vi "Dashboard Push.vi"() -> ()   [LabVIEW 2018]
uses:
  <vilib>/Rock Robotics/WPI/Joystick/WPI_JoystickDevRef.ctl
  <vilib>/Rock Robotics/WPI/Joystick/WPI_JoystickDeviceEnum.ctl
  b7084bc7-1634-490a-a06e-4582ec5dc279.vi
  Robot States.vi
  <vilib>/Rock Robotics/Network Tables/NT Write Boolean.vi
  Sensor Readings.vi
  Robot Global Data.vi
panel:
  in  "Joystick 0 Ref":T1
  in  "Joystick 1 Ref":T1
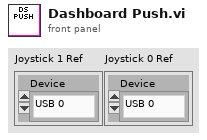
[diagram p1: front panel]
types:
  T1 = typedef "WPI_JoystickDevRef.ctl" = cluster{"Device":T2}
  T2 = typedef "WPI_JoystickDeviceEnum.ctl" = enum16{"USB 0", "USB 1", "USB 2", "USB 3", "USB 4", "USB 5"}
  T3 = cluster{"[0]":bool, "[1]":bool, "[2]":bool, "[3]":bool, "[4]":bool, "[5]":bool, "[6]":bool}
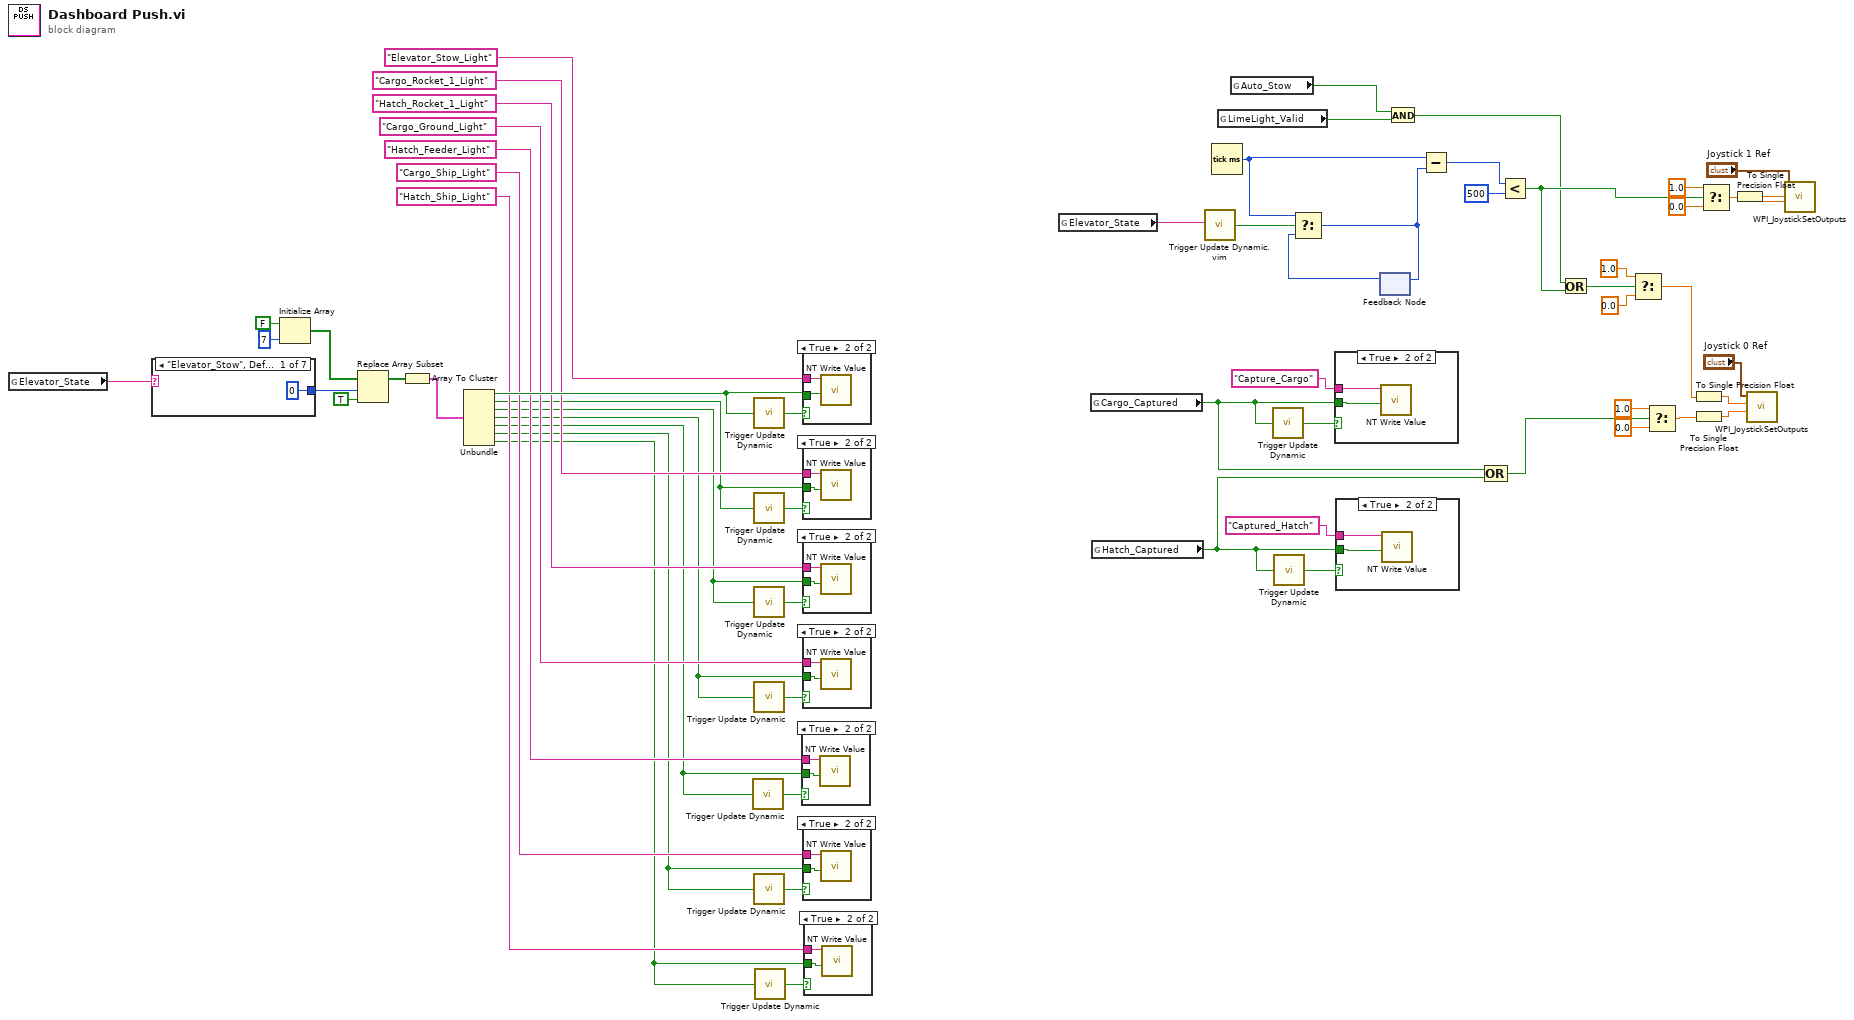
[diagram p0: block diagram]
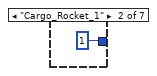
[diagram p11: hidden frame]
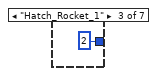
[diagram p12: hidden frame]
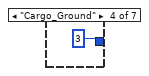
[diagram p13: hidden frame]
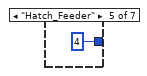
[diagram p14: hidden frame]
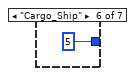
[diagram p15: hidden frame]
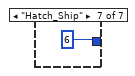
[diagram p16: hidden frame]
diagram:
  n1 = global read "Robot States.vi" "Elevator_State"() -> (w34:string)
  n2 = case shown="\"Elevator_Stow\", Default" w34 {
    tunnel: [0 1 2 3 4 5 6] -> w59
    frame "Elevator_Stow", Default {
    }
    frame "Cargo_Rocket_1" {
    }
    frame "Hatch_Rocket_1" {
    }
    frame "Cargo_Ground" {
    }
    frame "Hatch_Feeder" {
    }
    frame "Cargo_Ship" {
    }
    frame "Hatch_Ship" {
    }
  }
  n3 = Initialize Array(FALSE, 7 ("dimension size")) -> (w60:bool[])
  n4 = Replace Array Subset(array=w60, new element=TRUE ("new element/subarray"), index=w59) -> (w57:bool[])
  n5 = Array To Cluster(array=w57) -> (cluster=w35:T3)
  n6 = Unbundle(w35) -> ("[0]"=w55:bool, "[1]"=w41:bool, "[2]"=w40:bool, "[3]"=w39:bool, "[4]"=w38:bool, "[5]"=w37:bool, "[6]"=w36:bool)
  n7 = call "Trigger Update Dynamic.vi"("Trigger"=w38) -> ("Update"=w51:bool)
  n8 = call "Trigger Update Dynamic.vi"("Trigger"=w55) -> ("Update"=w56:bool)
  n9 = call "Trigger Update Dynamic.vi"("Trigger"=w41) -> ("Update"=w53:bool)
  n10 = call "Trigger Update Dynamic.vi"("Trigger"=w40) -> ("Update"=w52:bool)
  n11 = call "Trigger Update Dynamic.vi"("Trigger"=w39) -> ("Update"=w50:bool)
  n12 = call "Trigger Update Dynamic.vi"("Trigger"=w37) -> ("Update"=w49:bool)
  n13 = call "Trigger Update Dynamic.vi"("Trigger"=w36) -> ("Update"=w48:bool)
  n14 = case shown="True" w51 {
    tunnel: "Hatch_Feeder_Light" -> [_ w71]
    tunnel: w38 -> [_ w70]
    frame False {
    }
    frame True {
      n15 = call-poly <vilib>:"NT Write Value.vi"("Boolean"=w70, "Name"=w71) -> ()  [unwired: 9 in, 1 out]
    }
  }
  n16 = case shown="True" w56 {
    tunnel: w55 -> [_ w73]
    tunnel: "Elevator_Stow_Light" -> [_ w72]
    frame False {
    }
    frame True {
      n17 = call-poly <vilib>:"NT Write Value.vi"("Boolean"=w73, "Name"=w72) -> ()  [unwired: 9 in, 1 out]
    }
  }
  n18 = case shown="True" w53 {
    tunnel: "Cargo_Rocket_1_Light" -> [_ w75]
    tunnel: w41 -> [_ w74]
    frame False {
    }
    frame True {
      n19 = call-poly <vilib>:"NT Write Value.vi"("Boolean"=w74, "Name"=w75) -> ()  [unwired: 9 in, 1 out]
    }
  }
  n20 = case shown="True" w52 {
    tunnel: "Hatch_Rocket_1_Light" -> [_ w77]
    tunnel: w40 -> [_ w76]
    frame False {
    }
    frame True {
      n21 = call-poly <vilib>:"NT Write Value.vi"("Boolean"=w76, "Name"=w77) -> ()  [unwired: 9 in, 1 out]
    }
  }
  n22 = case shown="True" w50 {
    tunnel: "Cargo_Ground_Light" -> [_ w79]
    tunnel: w39 -> [_ w78]
    frame False {
    }
    frame True {
      n23 = call-poly <vilib>:"NT Write Value.vi"("Boolean"=w78, "Name"=w79) -> ()  [unwired: 9 in, 1 out]
    }
  }
  n24 = case shown="True" w49 {
    tunnel: "Cargo_Ship_Light" -> [_ w81]
    tunnel: w37 -> [_ w80]
    frame False {
    }
    frame True {
      n25 = call-poly <vilib>:"NT Write Value.vi"("Boolean"=w80, "Name"=w81) -> ()  [unwired: 9 in, 1 out]
    }
  }
  n26 = case shown="True" w48 {
    tunnel: "Hatch_Ship_Light" -> [_ w83]
    tunnel: w36 -> [_ w82]
    frame False {
    }
    frame True {
      n27 = call-poly <vilib>:"NT Write Value.vi"("Boolean"=w82, "Name"=w83) -> ()  [unwired: 9 in, 1 out]
    }
  }
  n28 = global read "Robot States.vi" "Elevator_State"() -> (w33:string)
  n29 = global read "Sensor Readings.vi" "Cargo_Captured"() -> (w14:bool)
  n30 = global read "Sensor Readings.vi" "Hatch_Captured"() -> (w13:bool)
  n31 = call "Trigger Update Dynamic.vim"("Trigger"=w33) -> ("Update"=w32:bool)
  n32 = Tick Count (ms)() -> (millisecond timer value=w30:u32)
  n33 = global read "Sensor Readings.vi" "LimeLight_Valid"() -> (w2:bool)
  n34 = global read "Robot States.vi" "Auto_Stow"() -> (w3:bool)
  n35 = call "Trigger Update Dynamic.vi"("Trigger"=w14) -> ("Update"=w18:bool)
  n36 = call "Trigger Update Dynamic.vi"("Trigger"=w13) -> ("Update"=w16:bool)
  n37 = case shown="True" w18 {
    tunnel: "Capture_Cargo" ("Name") -> [_ w85]
    tunnel: w14 -> [_ w84]
    frame False {
    }
    frame True {
      n38 = call-poly <vilib>:"NT Write Value.vi"("Boolean"=w84, "Name"=w85) -> ()  [unwired: 9 in, 1 out]
    }
  }
  n39 = case shown="True" w16 {
    tunnel: "Captured_Hatch" ("Name") -> [_ w87]
    tunnel: w13 -> [_ w86]
    frame False {
    }
    frame True {
      n40 = call-poly <vilib>:"NT Write Value.vi"("Boolean"=w86, "Name"=w87) -> ()  [unwired: 9 in, 1 out]
    }
  }
  n41 = feedback #1() -> (w31:u32)  [unwired: 1 in]
  n42 = Select(t=w30, s=w32, f=w31) -> (s? t:f=w29:u32)
  n43 = feedback-in #1(w29) -> ()
  n44 = And(x=w3, y=w2) -> (x .and. y?=w1:bool)
  n45 = Subtract(x=w30, y=w29) -> (x-y=w28:u32)
  n46 = Compound Arithmetic op=OR(w14, w13) -> (w12:bool)
  n47 = Less?(x=w28, y=u32 500) -> (x < y?=w11:bool)
  n48 = Or(x=w1, y=w11) -> (x .or. y?=w9:bool)
  n49 = Select(t=1.0, s=w9, f=0.0) -> (s? t:f=w5:dbl)
  n50 = Select(t=1.0, s=w12, f=0.0) -> (s? t:f=w20:dbl)
  n51 = To Single Precision Float(number=w5) -> (single precision float=w6:sgl)
  n52 = To Single Precision Float(number=w20) -> (single precision float=w7:sgl)
  n53 = Select(t=1.0, s=w11, f=0.0) -> (s? t:f=w24:dbl)
  n54 = To Single Precision Float(number=w24) -> (single precision float=w19:sgl)
  n55 = call <vilib>:"WPI_JoystickSetOutputs.vi"("Right Rumble"=w7, "Left Rumble"=w6, "JoystickDevRef"="Joystick 0 Ref") -> ()  [unwired: 7 in, 2 out]
  n56 = call <vilib>:"WPI_JoystickSetOutputs.vi"("Right Rumble"=w19, "Left Rumble"=w19, "JoystickDevRef"="Joystick 1 Ref") -> ()  [unwired: 7 in, 2 out]
